vi "Autonomous Independent.vi"() -> ()   [LabVIEW 2014]
doc: "This VI is called when autonomous begins, and will automatically be terminated when autonomous ends. You can carry out timed or sensor driven robot movement independently without needing to return to the caller."
uses:
  Robot Global Data.vi
  <vilib>/Rock Robotics/WPI/RobotDrive/WPI_RobotDriveMecanumDrive_Cartesian.vi
  <vilib>/Rock Robotics/Network Tables/SD Write Numeric Array.vi
panel:
  out "Current Movement, for debugging":T1 {"Z Joystick Value" scale=-1.0..1.0; "Y Joystick Value" scale=1.0..-1.0; "X Joystick Value" scale=-1.0..1.0}
  in  "Array of robot movements":T2(array[cluster]) {"Z Joystick Value" scale=-1.0..1.0; "Y Joystick Value" scale=1.0..-1.0; "X Joystick Value" scale=-1.0..1.0}
  # "Be sure to right-click and choose Data Operations>>Make Current Value default if you want to save the array values with the VI"
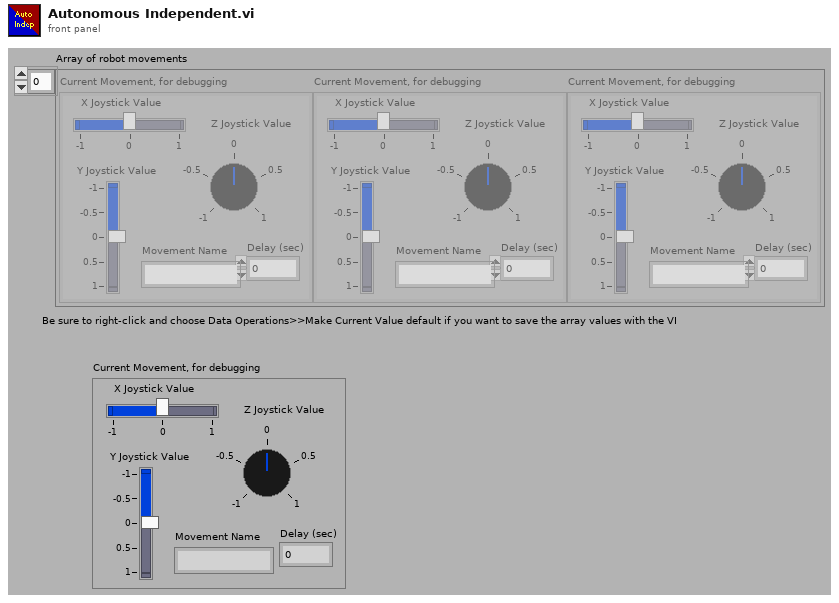
[diagram p1: front panel]
types:
  T1 = cluster{"X Joystick Value":dbl, "Y Joystick Value":dbl, "Z Joystick Value":dbl, "Delay (sec)":dbl, "Movement Name":string}
  T2 = cluster{"X Joystick Value":dbl, "Y Joystick Value":dbl, "Z Joystick Value":dbl, "Delay (sec)":dbl, "Movement Name":string}[]
  T3 = cluster{"Time to Start":dbl, "Action":enum16{"Stop", "Drive Forward", "Drive Backwards", "Turn Right", "Turn Left", "Tote Up", "Tote Down", "Doors Open", "Doors Close", "Claw Open", "Claw Close", "Claw Up", "Claw Down", "Infeed In", "Infeed Out", "Infeed Off"}}[]
  T4 = typedef "WPI_RobotDriveDevRef.ctl" = cluster{"DevStatus":errorcluster, "Motors[]":T5[], "Square Inputs":bool, "Max Output":dbl}
  T5 = typedef "WPI_MotorControlDeviceRef.ctl" = cluster{"DeviceStatus":errorcluster, "Type":T6, "PWM":cluster{"Controller":T7, "PWM Channel":T8, "DeadBand":T9}, "CAN":cluster{"Device Number":u8, "Control Mode":T10, "Semaphore":T11, "Max Vout":dbl, "TalonSRX Control Mode":T12}, "Invert":bool, "TransformRef":T13, "InvTransformRef":T13}
  T6 = typedef "WPI_MotorControlType.ctl" = enum16{"PWM", "CAN", "CANTalonSRX"}
  T7 = typedef "FPGA_TypedefDigitalModule.ctl" = enum16{"Controller 1"}
  T8 = typedef "FPGA_DIOPWMChannel.ctl" = enum8{"PWM 0", "PWM 1", "PWM 2", "PWM 3", "PWM 4", "PWM 5", "PWM 6", "PWM 7", "PWM 8", "PWM 9", "PWM MXP 0", "PWM MXP 1", "PWM MXP 2", "PWM MXP 3", "PWM MXP 4", "PWM MXP 5", "PWM MXP 6", "PWM MXP 7", "PWM MXP 8", "PWM MXP 9", "Invalid"}
  T9 = typedef "WPI_PWMDeadband.ctl" = cluster{"Name":string, "maxPositivePwm":i32, "minPositivePwm":i32, "centerPwm":i32, "maxNegativePwm":i32, "minNegativePwm":i32, "angularRange":u16}
  T10 = typedef "WPI_CANJaguar_ControlMode.ctl" = enum8{"Percent VBus", "Current", "Speed", "Position", "Voltage"}
  T11 = typedef "Semaphore RefNum" = refnum<k1>
  T12 = typedef "WPI_CANTalonSRX_APIControlMode.ctl" = enum8{"Percent VBus", "Speed", "Position", "Slave", "Unchanged / Invalid"}
  T13 = typedef "WPI_PWMTransform_ConPane.ctl" = refnum<vi>
  T14 = cluster{"Motor Speed":dbl, "Grabber":bool, "Go Up a Level":bool, "Go Down a Level":bool}
  T15 = cluster{"Lifter":bool, "Right Infeed":enum16{"Off", "Forward", "Reverse"}, "Left Infeed":enum16{"Off", "Forward", "Reverse"}}
  T16 = enum16{"Stop", "Drive Forward", "Drive Backwards", "Turn Right", "Turn Left", "Tote Up", "Tote Down", "Doors Open", "Doors Close", "Claw Open", "Claw Close", "Claw Up", "Claw Down", "Infeed In", "Infeed Out", "Infeed Off"}
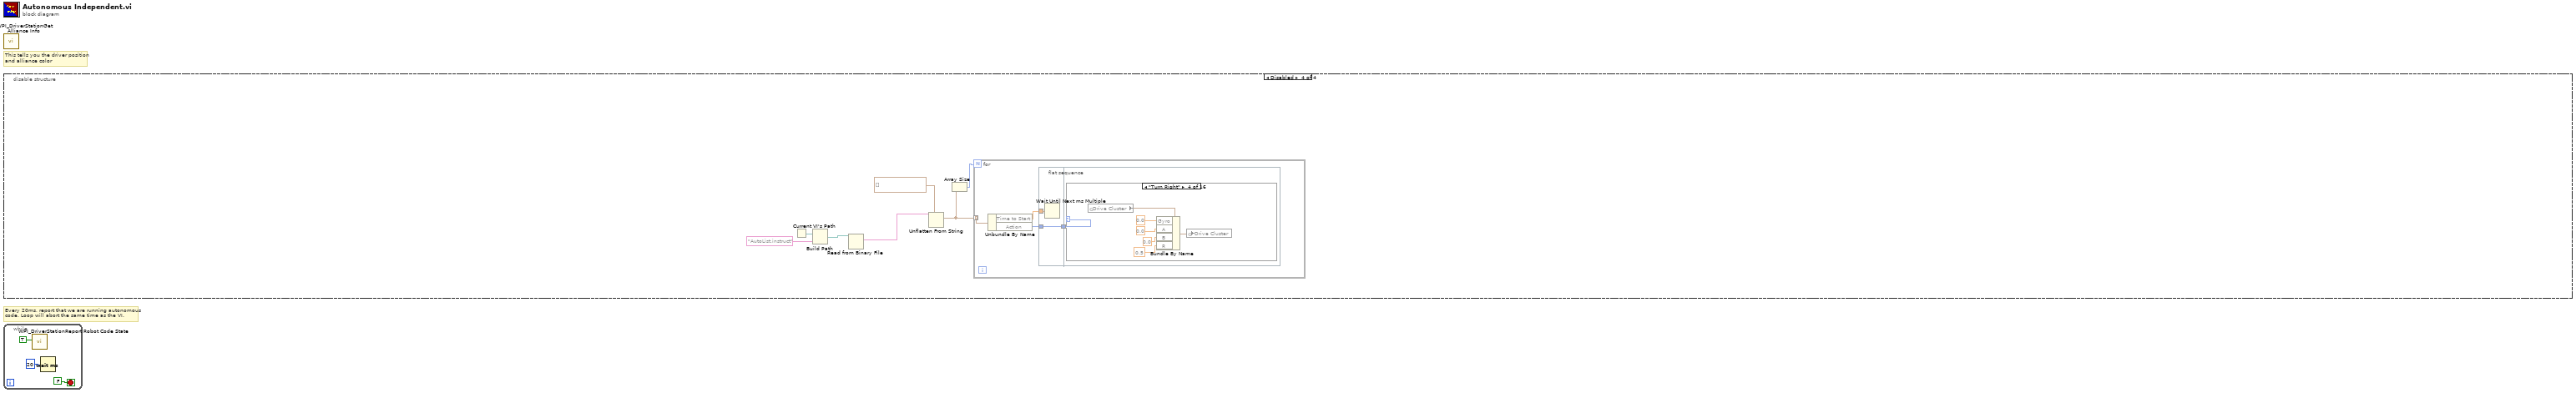
[diagram p0: block diagram]
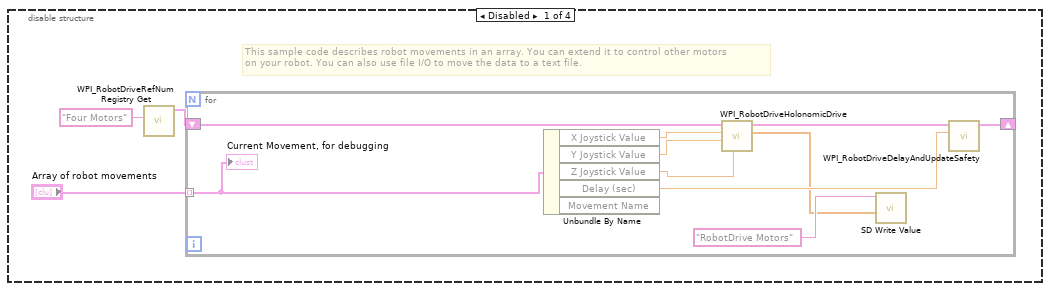
[diagram p2: hidden frame]
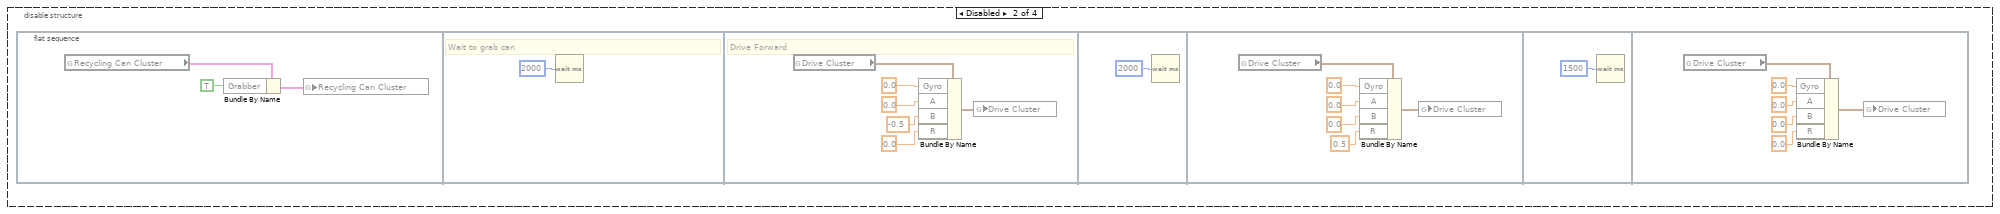
[diagram p3: hidden frame]
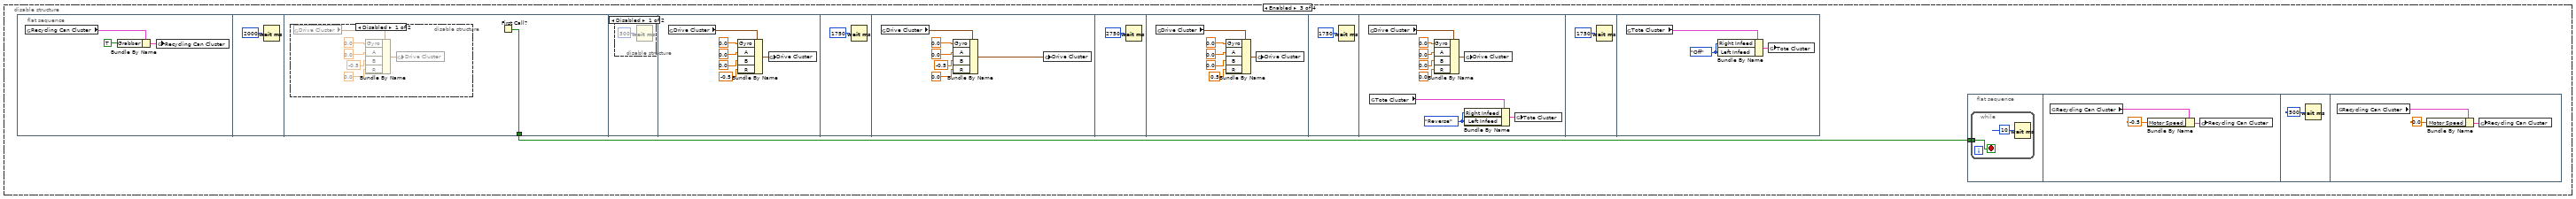
[diagram p4: hidden frame]
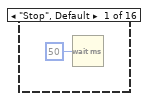
[diagram p7: hidden frame]
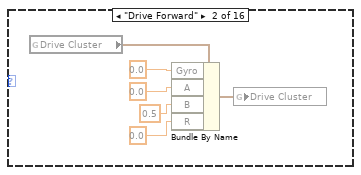
[diagram p8: hidden frame]
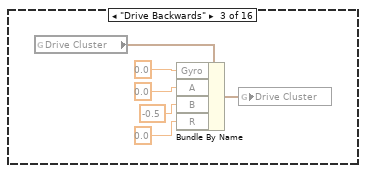
[diagram p9: hidden frame]
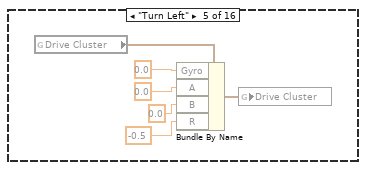
[diagram p10: hidden frame]
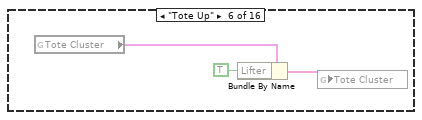
[diagram p11: hidden frame]
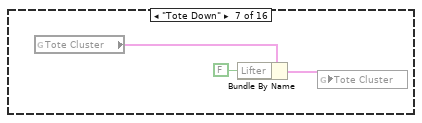
[diagram p12: hidden frame]
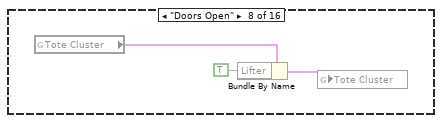
[diagram p13: hidden frame]
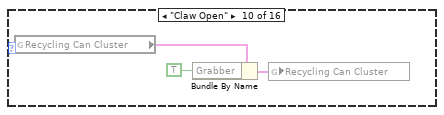
[diagram p15: hidden frame]
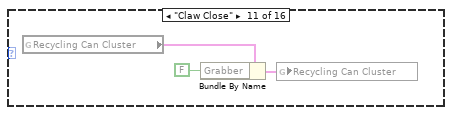
[diagram p16: hidden frame]
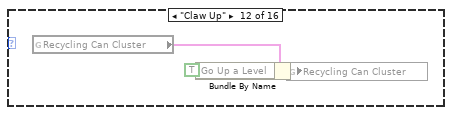
[diagram p17: hidden frame]
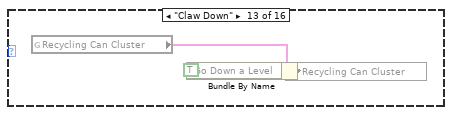
[diagram p18: hidden frame]
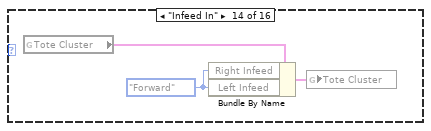
[diagram p19: hidden frame]
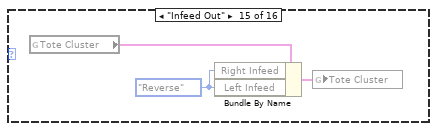
[diagram p20: hidden frame]
diagram:
  # "Every 20ms, report that we are running autonomous\ncode. Loop will abort the same time as the VI."
  # "This tells you the driver position\nand alliance color"
  n1 = call <vilib>:"WPI_DriverStationGet Alliance Info.vi"() -> ()  [unwired: 12 out]
  n2 = disable-structure shown="Disabled" {
    frame Disabled {
      # "This sample code describes robot movements in an array. You can extend it to control other motors\non your robot. You can also use file I/O to move the data to a text file."
      n3 = call <vilib>:"WPI_RobotDriveRefNum Registry Get.vi"("refnum name"="Four Motors") -> ("RobotDriveDevRef"=w2:T4)  [unwired: 1 in, 9 out]
      n4 = for {
        shift-right: [w10] -> _
        shift-left: w2 -> [w11]
        tunnel: "Array of robot movements" -> [w6] mode=indexing
        n5 = Unbundle By Name(w6) -> ("X Joystick Value"=w9:dbl, "Y Joystick Value"=w8:dbl, "Z Joystick Value"=w5:dbl, "Delay (sec)"=w7:dbl)  [unwired: 1 out]
        n6 = call-poly <vilib>:"WPI_RobotDriveHolonomicDrive.vi"("Rotation"=w5, "Y"=w8, "X"=w9, "RobotDriveDevRef"=w11) -> ("Motor Values"=w4:dbl[], "RobotDriveDevRef"=w12:T4)  [unwired: 5 in, 1 out]
        n7 = call-poly <vilib>:"SD Write Value.vi"("Numeric Array"=w4, "Name"="RobotDrive Motors") -> ()  [unwired: 8 in, 2 out]
        n8 = call <vilib>:"WPI_RobotDriveDelayAndUpdateSafety.vi"("Delay (s)"=w7, "RobotDriveDevRef"=w12) -> ("RobotDriveDevRef 2"=w10:T4)  [unwired: 8 in, 1 out]
        "Current Movement, for debugging" <- w6
      }
    }
    frame Disabled {
      n9 = flat-sequence {
        frame #0 {
          n10 = global read "Robot Global Data.vi" "Recycling Can Cluster"() -> (w15:T14)
          n11 = Bundle By Name(cluster=w15, "Grabber"=TRUE) -> (w14:T14)
          n12 = global write "Robot Global Data.vi" "Recycling Can Cluster"(w14) -> ()
        }
        frame #1 {
          # "Wait to grab can"
          n13 = Wait (ms)(milliseconds to wait=u32 2000) -> ()  [unwired: 1 out]
        }
        frame #2 {
          # "Drive Forward"
          n14 = global read "Robot Global Data.vi" "Drive Cluster"() -> (w23:cluster{"A":dbl, "B":dbl, "R":dbl, "Gyro":dbl})
          n15 = Bundle By Name(cluster=w23, "Gyro"=0.0, "A"=0.0, "B"=-0.5, "R"=0.0) -> (w22:cluster{"A":dbl, "B":dbl, "R":dbl, "Gyro":dbl})
          n16 = global write "Robot Global Data.vi" "Drive Cluster"(w22) -> ()
        }
        frame #3 {
          n17 = Wait (ms)(milliseconds to wait=u32 2000 ("millisecond multiple")) -> ()  [unwired: 1 out]
        }
        frame #4 {
          n18 = global read "Robot Global Data.vi" "Drive Cluster"() -> (w25:cluster{"A":dbl, "B":dbl, "R":dbl, "Gyro":dbl})
          n19 = Bundle By Name(cluster=w25, "Gyro"=0.0, "A"=0.0, "B"=0.0, "R"=0.5) -> (w26:cluster{"A":dbl, "B":dbl, "R":dbl, "Gyro":dbl})
          n20 = global write "Robot Global Data.vi" "Drive Cluster"(w26) -> ()
        }
        frame #5 {
          n21 = Wait (ms)(milliseconds to wait=u32 1500 ("millisecond multiple")) -> ()  [unwired: 1 out]
        }
        frame #6 {
          n22 = global read "Robot Global Data.vi" "Drive Cluster"() -> (w32:cluster{"A":dbl, "B":dbl, "R":dbl, "Gyro":dbl})
          n23 = Bundle By Name(cluster=w32, "Gyro"=0.0, "A"=0.0, "B"=0.0, "R"=0.0) -> (w33:cluster{"A":dbl, "B":dbl, "R":dbl, "Gyro":dbl})
          n24 = global write "Robot Global Data.vi" "Drive Cluster"(w33) -> ()
        }
      }
    }
    frame Enabled {
      n25 = flat-sequence {
        tunnel: [w53] -> w38
        frame #0 {
          n26 = global read "Robot Global Data.vi" "Recycling Can Cluster"() -> (w50:T14)
          n27 = Bundle By Name(cluster=w50, "Grabber"=TRUE) -> (w49:T14)
          n28 = global write "Robot Global Data.vi" "Recycling Can Cluster"(w49) -> ()
        }
        frame #1 {
          n29 = Wait (ms)(milliseconds to wait=u32 2000) -> ()  [unwired: 1 out]
        }
        frame #2 {
          n30 = disable-structure shown="Disabled" {
            frame Disabled {
              n31 = global read "Robot Global Data.vi" "Drive Cluster"() -> (w59:cluster{"A":dbl, "B":dbl, "R":dbl, "Gyro":dbl})
              n32 = Bundle By Name(cluster=w59, "Gyro"=0.0, "A"=0.0, "B"=-0.5, "R"=0.0) -> (w58:cluster{"A":dbl, "B":dbl, "R":dbl, "Gyro":dbl})
              n33 = global write "Robot Global Data.vi" "Drive Cluster"(w58) -> ()
            }
            frame Enabled {
            }
          }
          n34 = First Call?() -> (First Call?: T/F=w53:bool)
        }
        frame #3 {
          n35 = disable-structure shown="Disabled" {
            frame Disabled {
              n36 = Wait (ms)(milliseconds to wait=u32 300) -> ()  [unwired: 1 out]
            }
            frame Enabled {
            }
          }
        }
        frame #4 {
          n37 = global read "Robot Global Data.vi" "Drive Cluster"() -> (w62:cluster{"A":dbl, "B":dbl, "R":dbl, "Gyro":dbl})
          n38 = Bundle By Name(cluster=w62, "Gyro"=0.0, "A"=0.0, "B"=0.0, "R"=-0.5) -> (w63:cluster{"A":dbl, "B":dbl, "R":dbl, "Gyro":dbl})
          n39 = global write "Robot Global Data.vi" "Drive Cluster"(w63) -> ()
        }
        frame #5 {
          n40 = Wait (ms)(milliseconds to wait=u32 1750 ("millisecond multiple")) -> ()  [unwired: 1 out]
        }
        frame #6 {
          n41 = global read "Robot Global Data.vi" "Drive Cluster"() -> (w68:cluster{"A":dbl, "B":dbl, "R":dbl, "Gyro":dbl})
          n42 = Bundle By Name(cluster=w68, "Gyro"=0.0, "A"=0.0, "B"=-0.5, "R"=0.0) -> (w69:cluster{"A":dbl, "B":dbl, "R":dbl, "Gyro":dbl})
          n43 = global write "Robot Global Data.vi" "Drive Cluster"(w69) -> ()
        }
        frame #7 {
          n44 = Wait (ms)(milliseconds to wait=u32 2750 ("millisecond multiple")) -> ()  [unwired: 1 out]
        }
        frame #8 {
          n45 = global read "Robot Global Data.vi" "Drive Cluster"() -> (w75:cluster{"A":dbl, "B":dbl, "R":dbl, "Gyro":dbl})
          n46 = Bundle By Name(cluster=w75, "Gyro"=0.0, "A"=0.0, "B"=0.0, "R"=0.5) -> (w76:cluster{"A":dbl, "B":dbl, "R":dbl, "Gyro":dbl})
          n47 = global write "Robot Global Data.vi" "Drive Cluster"(w76) -> ()
        }
        frame #9 {
          n48 = Wait (ms)(milliseconds to wait=u32 1750 ("millisecond multiple")) -> ()  [unwired: 1 out]
        }
        frame #10 {
          w82 = enum16{"Off", "Forward", "Reverse"}."Reverse" ("Right Infeed")
          n49 = global read "Robot Global Data.vi" "Drive Cluster"() -> (w90:cluster{"A":dbl, "B":dbl, "R":dbl, "Gyro":dbl})
          n50 = global read "Robot Global Data.vi" "Tote Cluster"() -> (w83:T15)
          n51 = Bundle By Name(cluster=w90, "Gyro"=0.0, "A"=0.0, "B"=0.0, "R"=0.0) -> (w89:cluster{"A":dbl, "B":dbl, "R":dbl, "Gyro":dbl})
          n52 = global write "Robot Global Data.vi" "Drive Cluster"(w89) -> ()
          n53 = Bundle By Name(cluster=w83, "Right Infeed"=w82, "Left Infeed"=w82) -> (w84:T15)
          n54 = global write "Robot Global Data.vi" "Tote Cluster"(w84) -> ()
        }
        frame #11 {
          n55 = Wait (ms)(milliseconds to wait=u32 1750 ("millisecond multiple")) -> ()  [unwired: 1 out]
        }
        frame #12 {
          w92 = enum16{"Off", "Forward", "Reverse"}."Off" ("Right Infeed")
          n56 = global read "Robot Global Data.vi" "Tote Cluster"() -> (w93:T15)
          n57 = Bundle By Name(cluster=w93, "Right Infeed"=w92, "Left Infeed"=w92) -> (w94:T15)
          n58 = global write "Robot Global Data.vi" "Tote Cluster"(w94) -> ()
        }
      }
      n59 = flat-sequence {
        tunnel: w38 -> [w39]
        frame #0 {
          n60 = while {
            tunnel: w39 -> [w41]
            stop <- w41 stop-if-true
            n61 = Wait (ms)(milliseconds to wait=u32 10) -> ()  [unwired: 1 out]
          }
        }
        frame #1 {
          n62 = global read "Robot Global Data.vi" "Recycling Can Cluster"() -> (w43:T14)
          n63 = Bundle By Name(cluster=w43, "Motor Speed"=-0.5) -> (w42:T14)
          n64 = global write "Robot Global Data.vi" "Recycling Can Cluster"(w42) -> ()
        }
        frame #2 {
          n65 = Wait (ms)(milliseconds to wait=u32 500) -> ()  [unwired: 1 out]
        }
        frame #3 {
          n66 = global read "Robot Global Data.vi" "Recycling Can Cluster"() -> (w47:T14)
          n67 = Bundle By Name(cluster=w47, "Motor Speed"=0.0) -> (w46:T14)
          n68 = global write "Robot Global Data.vi" "Recycling Can Cluster"(w46) -> ()
        }
      }
    }
    frame Disabled {
      n69 = Current VI's Path() -> (path=w98:path)
      n70 = Build Path(base path=w98, name or relative path="AutoList.instruct") -> (appended path=w100:path)
      n71 = Read from Binary File(11:w100) -> (2:w97:string)  [unwired: 5 in, 3 out]
      n72 = Unflatten From String(type=T3 [] ("Actions"), binary string=w97) -> (value=w95:T3)  [unwired: 3 in, 2 out]
      n73 = Array Size(array=w95) -> (size(s)=w96:i32)
      n74 = for {
        N: w96 -> [_]
        tunnel: w95 -> [w105] mode=indexing
        n75 = Unbundle By Name(w105) -> ("Time to Start"=w104:dbl, "Action"=w102:T16)
        n76 = flat-sequence {
          tunnel: w104 -> [w107]
          tunnel: [w106] -> w103
          tunnel: w102 -> [w106]
          tunnel: w103 -> [w108]
          frame #0 {
            n77 = Wait Until Next ms Multiple(millisecond multiple=w107) -> ()  [unwired: 1 out]
          }
          frame #1 {
            n78 = case shown="\"Turn Right\"" w108 {
              frame "Stop", Default {
                n79 = Wait (ms)(milliseconds to wait=u32 50) -> ()  [unwired: 1 out]
              }
              frame "Drive Forward" {
                n80 = global read "Robot Global Data.vi" "Drive Cluster"() -> (w115:cluster{"A":dbl, "B":dbl, "R":dbl, "Gyro":dbl})
                n81 = Bundle By Name(cluster=w115, "Gyro"=0.0, "A"=0.0, "B"=0.5, "R"=0.0) -> (w114:cluster{"A":dbl, "B":dbl, "R":dbl, "Gyro":dbl})
                n82 = global write "Robot Global Data.vi" "Drive Cluster"(w114) -> ()
              }
              frame "Drive Backwards" {
                n83 = global read "Robot Global Data.vi" "Drive Cluster"() -> (w116:cluster{"A":dbl, "B":dbl, "R":dbl, "Gyro":dbl})
                n84 = Bundle By Name(cluster=w116, "Gyro"=0.0, "A"=0.0, "B"=-0.5, "R"=0.0) -> (w117:cluster{"A":dbl, "B":dbl, "R":dbl, "Gyro":dbl})
                n85 = global write "Robot Global Data.vi" "Drive Cluster"(w117) -> ()
              }
              frame "Turn Right" {
                n86 = global read "Robot Global Data.vi" "Drive Cluster"() -> (w122:cluster{"A":dbl, "B":dbl, "R":dbl, "Gyro":dbl})
                n87 = Bundle By Name(cluster=w122, "Gyro"=0.0, "A"=0.0, "B"=0.0, "R"=0.5) -> (w123:cluster{"A":dbl, "B":dbl, "R":dbl, "Gyro":dbl})
                n88 = global write "Robot Global Data.vi" "Drive Cluster"(w123) -> ()
              }
              frame "Turn Left" {
                n89 = global read "Robot Global Data.vi" "Drive Cluster"() -> (w128:cluster{"A":dbl, "B":dbl, "R":dbl, "Gyro":dbl})
                n90 = Bundle By Name(cluster=w128, "Gyro"=0.0, "A"=0.0, "B"=0.0, "R"=-0.5) -> (w129:cluster{"A":dbl, "B":dbl, "R":dbl, "Gyro":dbl})
                n91 = global write "Robot Global Data.vi" "Drive Cluster"(w129) -> ()
              }
              frame "Tote Up" {
                n92 = global read "Robot Global Data.vi" "Tote Cluster"() -> (w135:T15)
                n93 = Bundle By Name(cluster=w135, "Lifter"=TRUE) -> (w136:T15)
                n94 = global write "Robot Global Data.vi" "Tote Cluster"(w136) -> ()
              }
              frame "Tote Down" {
                n95 = global read "Robot Global Data.vi" "Tote Cluster"() -> (w138:T15)
                n96 = Bundle By Name(cluster=w138, "Lifter"=FALSE) -> (w139:T15)
                n97 = global write "Robot Global Data.vi" "Tote Cluster"(w139) -> ()
              }
              frame "Doors Open" {
                n98 = global read "Robot Global Data.vi" "Tote Cluster"() -> (w141:T15)
                n99 = Bundle By Name(cluster=w141, "Lifter"=TRUE) -> (w140:T15)
                n100 = global write "Robot Global Data.vi" "Tote Cluster"(w140) -> ()
              }
              frame "Doors Close" {
              }
              frame "Claw Open" {
                n101 = global read "Robot Global Data.vi" "Recycling Can Cluster"() -> (w144:T14)
                n102 = Bundle By Name(cluster=w144, "Grabber"=TRUE) -> (w143:T14)
                n103 = global write "Robot Global Data.vi" "Recycling Can Cluster"(w143) -> ()
              }
              frame "Claw Close" {
                n104 = global read "Robot Global Data.vi" "Recycling Can Cluster"() -> (w147:T14)
                n105 = Bundle By Name(cluster=w147, "Grabber"=FALSE) -> (w148:T14)
                n106 = global write "Robot Global Data.vi" "Recycling Can Cluster"(w148) -> ()
              }
              frame "Claw Up" {
                n107 = global read "Robot Global Data.vi" "Recycling Can Cluster"() -> (w150:T14)
                n108 = Bundle By Name(cluster=w150, "Go Up a Level"=TRUE ("Grabber")) -> (w151:T14)
                n109 = global write "Robot Global Data.vi" "Recycling Can Cluster"(w151) -> ()
              }
              frame "Claw Down" {
                n110 = global read "Robot Global Data.vi" "Recycling Can Cluster"() -> (w153:T14)
                n111 = Bundle By Name(cluster=w153, "Go Down a Level"=TRUE ("Grabber")) -> (w154:T14)
                n112 = global write "Robot Global Data.vi" "Recycling Can Cluster"(w154) -> ()
              }
              frame "Infeed In" {
                w155 = enum16{"Off", "Forward", "Reverse"}."Forward" ("Right Infeed")
                n113 = global read "Robot Global Data.vi" "Tote Cluster"() -> (w156:T15)
                n114 = Bundle By Name(cluster=w156, "Right Infeed"=w155, "Left Infeed"=w155) -> (w157:T15)
                n115 = global write "Robot Global Data.vi" "Tote Cluster"(w157) -> ()
              }
              frame "Infeed Out" {
                w158 = enum16{"Off", "Forward", "Reverse"}."Reverse" ("Right Infeed")
                n116 = global read "Robot Global Data.vi" "Tote Cluster"() -> (w159:T15)
                n117 = Bundle By Name(cluster=w159, "Right Infeed"=w158, "Left Infeed"=w158) -> (w160:T15)
                n118 = global write "Robot Global Data.vi" "Tote Cluster"(w160) -> ()
              }
              frame "Infeed Off" {
                w163 = enum16{"Off", "Forward", "Reverse"}."Off" ("Right Infeed")
                n119 = global read "Robot Global Data.vi" "Tote Cluster"() -> (w162:T15)
                n120 = Bundle By Name(cluster=w162, "Right Infeed"=w163, "Left Infeed"=w163) -> (w161:T15)
                n121 = global write "Robot Global Data.vi" "Tote Cluster"(w161) -> ()
              }
            }
          }
        }
      }
    }
  }
  n122 = while {
    stop <- FALSE stop-if-true
    n123 = call <vilib>:"WPI_DriverStationReport Robot Code State.vi"("Autonomous"=TRUE) -> ()  [unwired: 10 in, 1 out]
    n124 = Wait (ms)(milliseconds to wait=u32 20) -> ()  [unwired: 1 out]
  }
